vi "Main.vi"() -> (0 "error out":errorcluster)   [LabVIEW 2020, in "Program.lvclass"]
uses:
  Program.lvclass
  BreakfastMenu_class/BreakfastMenu.lvclass
  DinnerMenu_class/DinnerMenu.lvclass
  Client_class/Client.lvclass
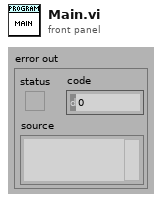
[diagram p1: front panel]
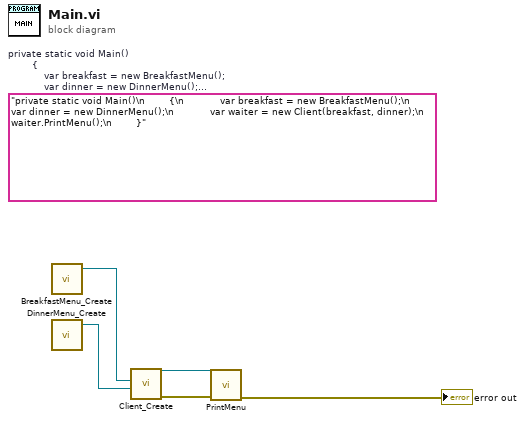
[diagram p0: block diagram]
diagram:
  (unwired) "private static void Main()\n        {\n            var breakfast = new BreakfastMenu();\n            var dinner = new DinnerMenu();\n            var waiter = new Client(breakfast, dinner);\n            waiter.PrintMenu();\n        }"  # private static void Main()         {             var breakfast = new BreakfastMenu();             var dinner = new DinnerMenu();             var waiter = new Client(breakfast, dinner);             waiter.PrintMenu();         }
  n1 = call "BreakfastMenu_Create.vi"() -> ("reference out"=w5:refnum<class "BreakfastMenu.lvclass">)  [unwired: 10 in, 1 out]
  n2 = call "DinnerMenu_Create.vi"() -> ("reference out"=w4:refnum<class "DinnerMenu.lvclass">)  [unwired: 10 in, 1 out]
  n3 = call "Client_Create.vi"("Dinner"=w4, "Breakfast"=w5) -> ("Error Out"=w2:errorcluster, "reference out"=w3:refnum<class "Client.lvclass">)  [unwired: 8 in]
  n4 = call-dynamic "PrintMenu.vi"("Error In"=w2, "reference in"=w3) -> ("Error Out"=→"error out":errorcluster)  [unwired: 8 in, 1 out]
